vi "Process.vi"(8 "error in":errorcluster, 11 "Inst.Xeryon-Rotator":refnum<class "Inst.Xeryon-Rotator.lvclass">) -> (0 "error out":errorcluster, 3 "Inst.Xeryon-Rotator out":refnum<class "Inst.Xeryon-Rotator.lvclass">)   [LabVIEW 2019, in "Inst.Xeryon-Rotator.lvclass"]
doc: "---------------------------------------------------------------\nJKI State Machine Objects™\nhttp://jki.net/state-machine-objects/\nCopyright (C) 2005-2015, JKI <info@jki.net>\nALL RIGHTS RESERVED"
uses:
  Inst.Xeryon-Rotator.lvclass
  C:/Program Files/National Instruments/LabVIEW 2019/user.lib/LevyLab/Instrument Framework/Instrument Types/Cryostat/Instrument.Cryostat.lvclass
  C:/Program Files/National Instruments/LabVIEW 2019/user.lib/LevyLab/Instrument Framework/Instrument/Instrument.lvclass
  C:/Program Files/National Instruments/LabVIEW 2019/vi.lib/JKI/JKI SMO/SMO/SMO.lvclass
  <userlib>/LevyLab/Instrument Framework/Instrument/Instrument.lvclass
  <userlib>/LevyLab/RemoteControl/RemoteControl/Typedefs/Message--Cluster.ctl
  <userlib>/LevyLab/RemoteControl/RemoteControl/RemoteControl.lvclass
  Typedefs/PrivateEvents--Inst.Xeryon-Rotator.MessageToProcess.ctl
  f3e0a8c3-f545-4415-8120-73ea4d9772d3.vi
  cbce47eb-2e04-4774-9aae-1c3eb2914706.vi
  <vilib>/JDP Science/JSONtext/JSONtext.lvlib
  828899be-930a-4dca-b584-bfe75166f4b0.vi
  Typedefs/Inst.Xeryon-Rotator.ScanState--Enum.ctl
  <userlib>/LevyLab/Debug/Debug.lvlib
  <userlib>/LevyLab/Instrument Framework/Instrument Types/Cryostat/Typedefs/setAngle--cluster.ctl
  <userlib>/LevyLab/Instrument Framework/Instrument Types/Cryostat/Instrument.Cryostat.lvclass
  <userlib>/LevyLab/Instrument Framework/Instrument/API/Instrument.sendMessageToProcess (variant).vi
  <vilib>/JKI/JKI SMO/SMO/SMO.lvclass
  bd7500a4-fca6-4b1e-8595-4df63a7e1bab.vi
panel:
  out "Data":string
  out "Status":string
  out "State History":string
  # "Instrument.Xeryon-Rotator"
  # "Xeryon-Rotator"
  # "For instructions on how to use the JKI State Machine Objects, examples and video tutorials, visit:\nhttp://jki.net/state-machine-objects/\n\nJKI State Machine Objects™\nhttp://jki.net/state-machine-objects/\nCopyright (C) 2005-2015, JKI <info@jki.net>\nALL RIGHTS RESERVED"
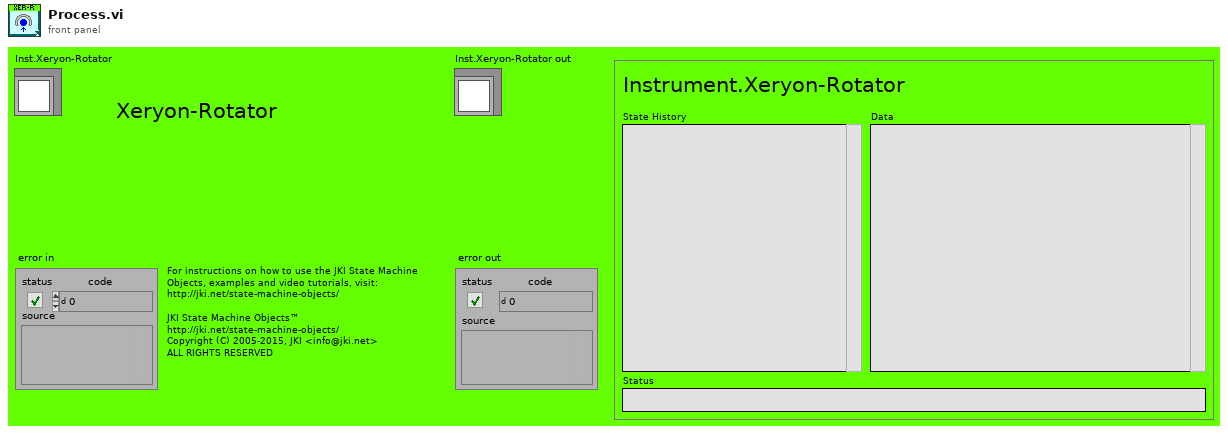
[diagram p1: front panel]
types:
  T1 = enum32{"invalid app kind", "Development System", "Run Time System", "Student Edition", "Embedded LabVIEW", "Evaluation", "Custom"}
  T2 = enum32{"Invalid", "Standard", "Closed", "Hidden", "Minimized", "Maximized"}
  T3 = typedef "Instrument.Cryostat.lvclass/setAngle--cluster.ctl" = cluster{"angle":dbl, "rate":dbl, "channel":i32}
  T4 = typedef "Inst.Xeryon-Rotator.lvclass/Inst.Xeryon-Rotator.ScanState--Enum.ctl" = enum16{"Scan Left", "Stop", "Scan Right", "Reset"}
  T5 = typedef "RemoteControl.lvlib/RemoteControl.lvclass/Message--Cluster.ctl" = cluster{"Command":string, "Data":variant, "ID":string, "error":errorcluster}
  T6 = typedef "Inst.Xeryon-Rotator.lvclass/PrivateEvents--Inst.Xeryon-Rotator.MessageToProcess.ctl" = cluster{"Message":T5}
  T7 = cluster{"Core":cluster{"Current VI Reference":refnum<vi>, "Close Panel on Exit?":bool, "Last Error":cluster{"error":errorcluster, "previous state":string, "remaining states":string}, "Shutdown?":bool}, "SMO":refnum<class "Inst.Xeryon-Rotator.lvclass">, "Running Step":i32, "sequence":string[], "MessageToProcess":T6}
  T8 = cluster{"Current VI Reference":refnum<vi>, "Close Panel on Exit?":bool, "Last Error":cluster{"error":errorcluster, "previous state":string, "remaining states":string}, "Shutdown?":bool}
  T9 = typedef "Debug.lvlib/Attribute.Debug.lvclass/DebugBehavior.ctl" = enum16{"Normal", "Debug"}
  T10 = typedef "SMO.lvclass/Protected Events.ctl" = cluster{"StopProcesses":refnum<user-event>, "AbortProcesses":refnum<user-event>, "Config Changed":refnum<user-event>, "Dependency":refnum<user-event>}
  T11 = cluster{"Encoder position [selected units]":dbl, "Desired Position [selected units]":dbl, "Status":string}
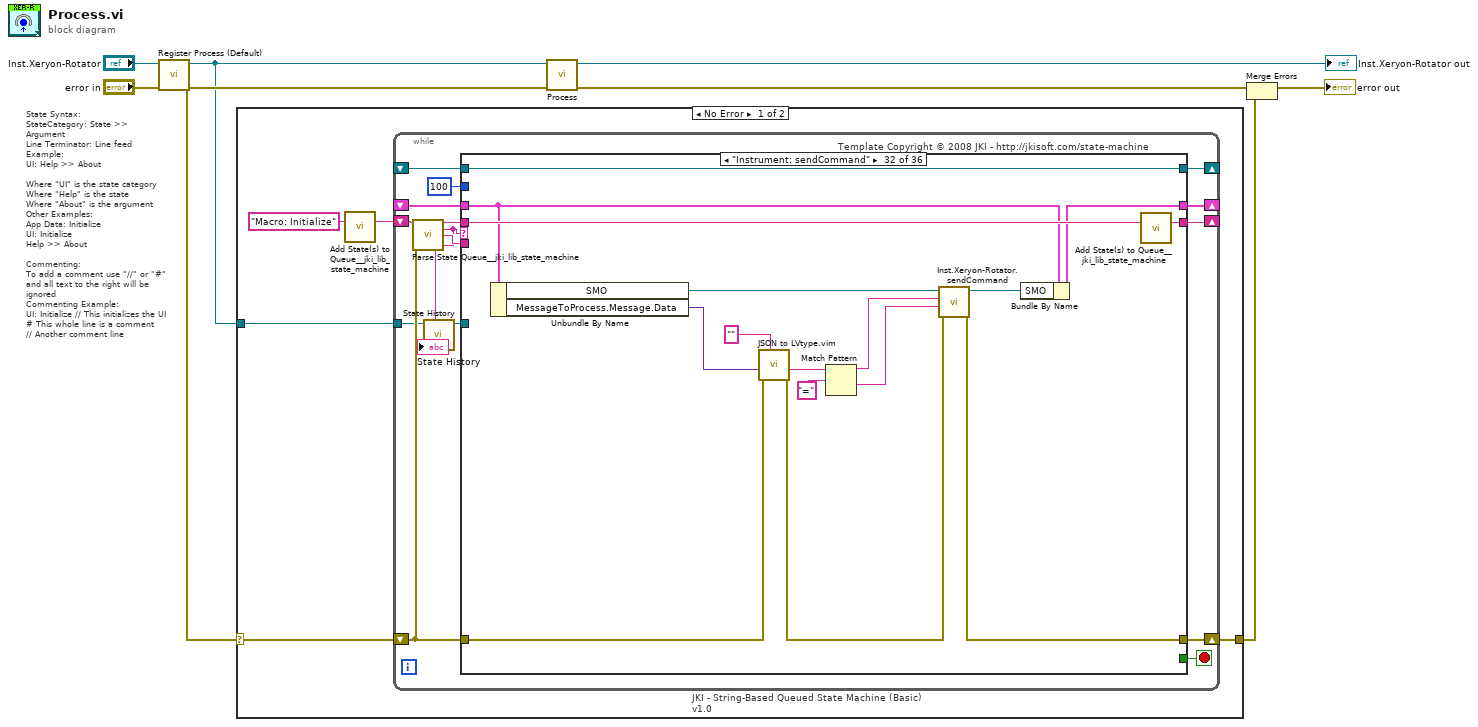
[diagram p0: block diagram]
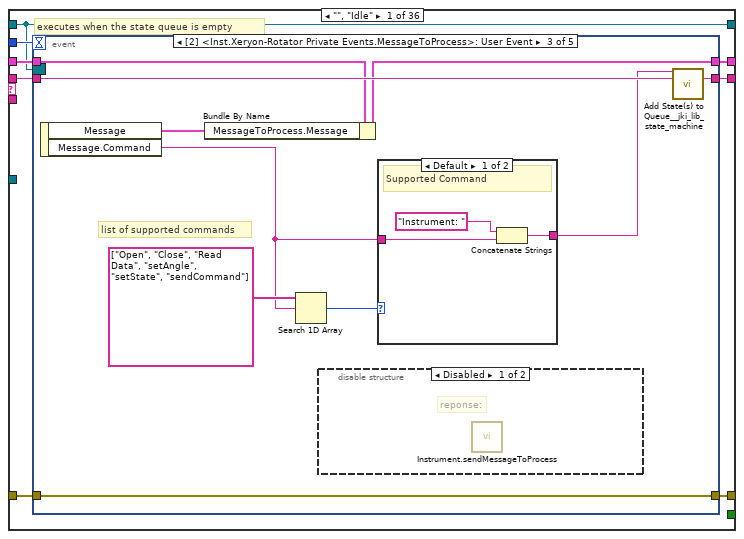
[diagram p2: hidden frame]
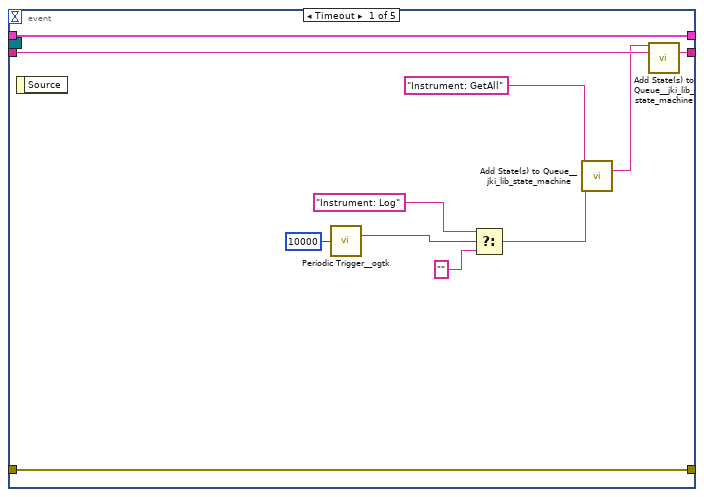
[diagram p3: hidden frame]
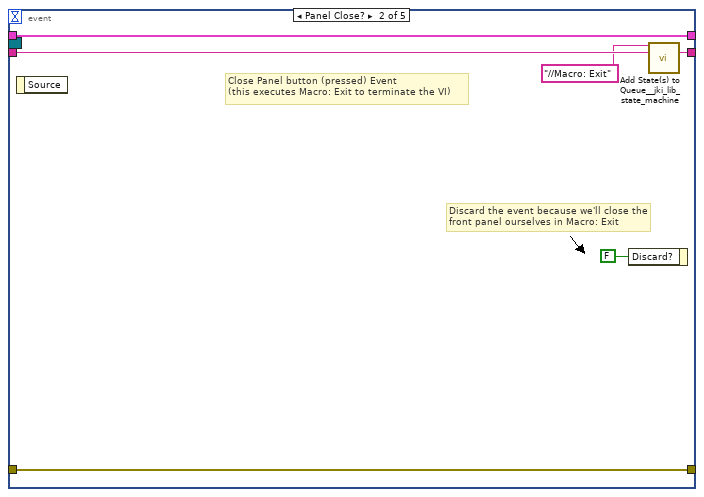
[diagram p4: hidden frame]
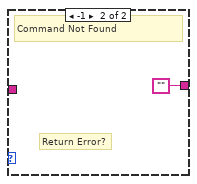
[diagram p6: hidden frame]
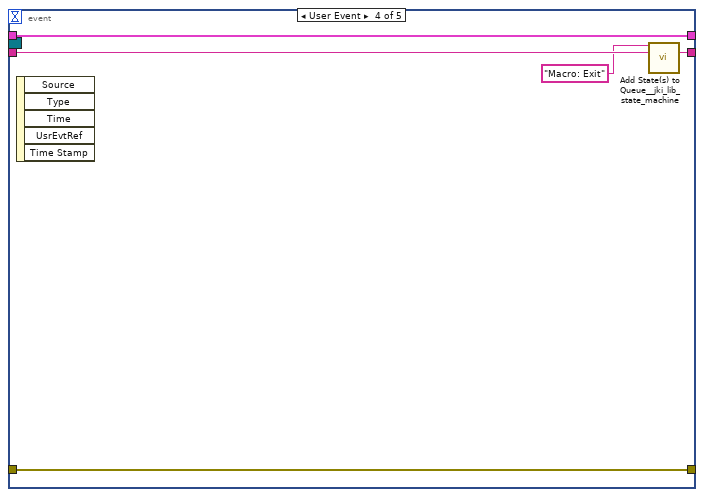
[diagram p7: hidden frame]
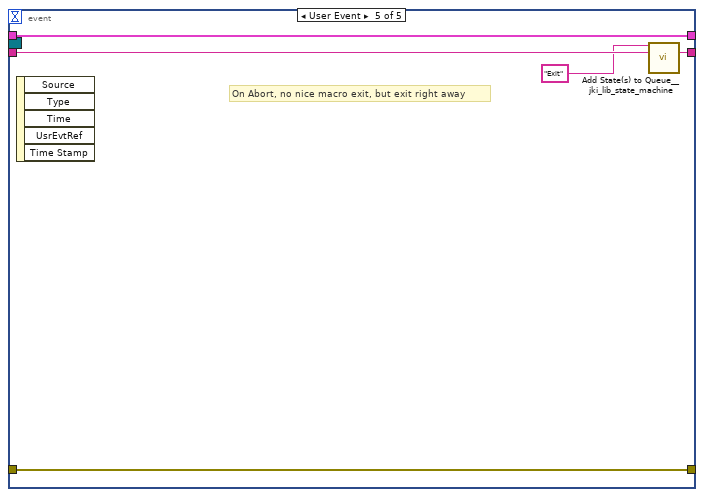
[diagram p8: hidden frame]
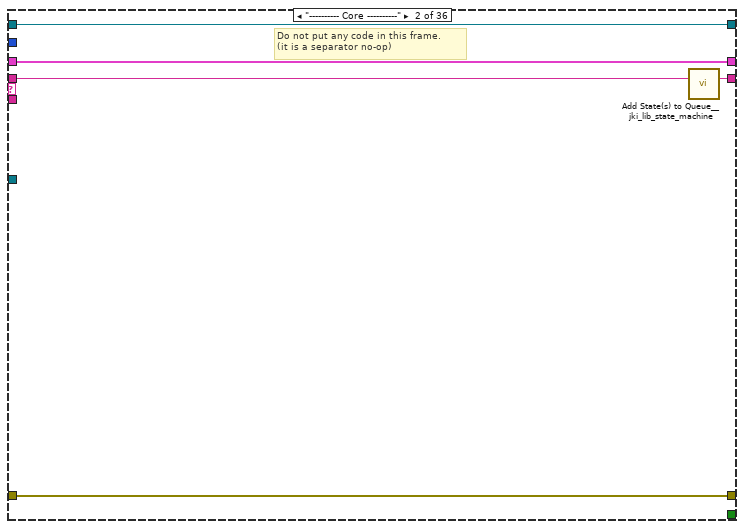
[diagram p9: hidden frame]
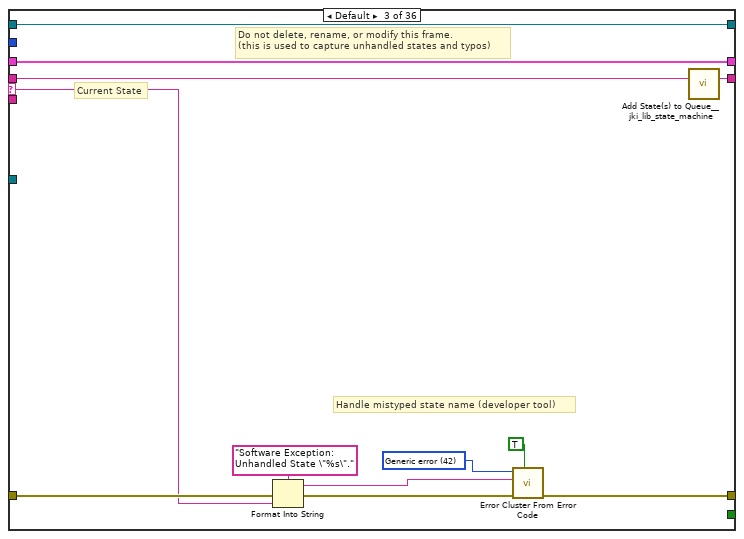
[diagram p10: hidden frame]
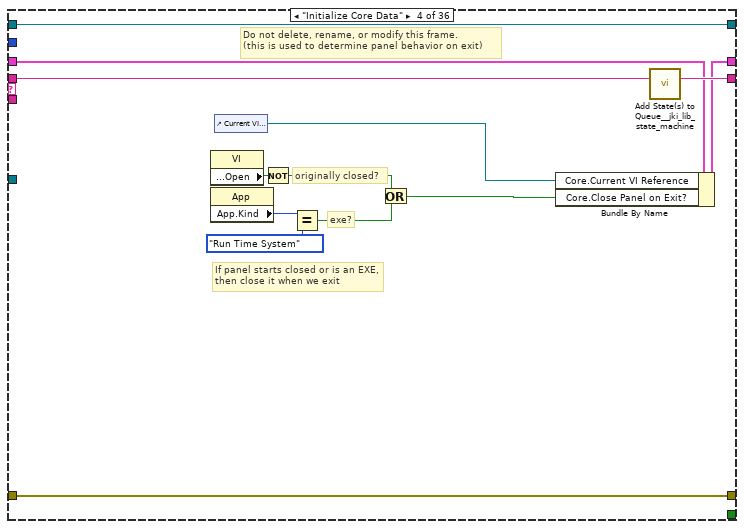
[diagram p11: hidden frame]
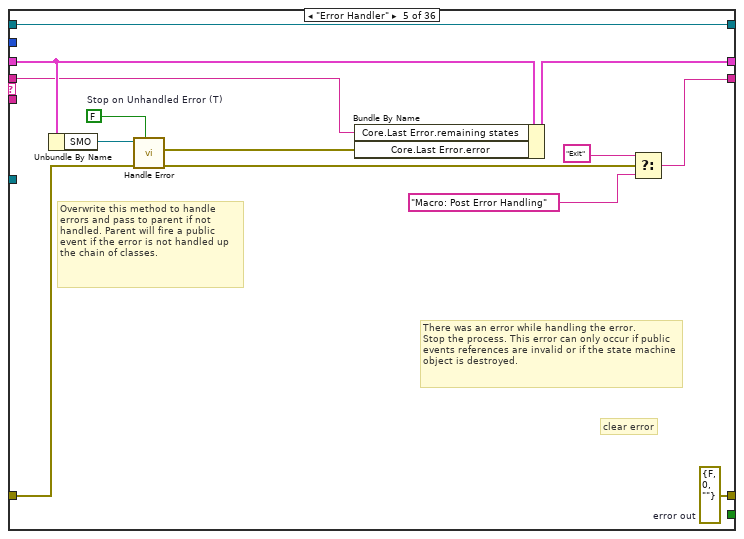
[diagram p12: hidden frame]
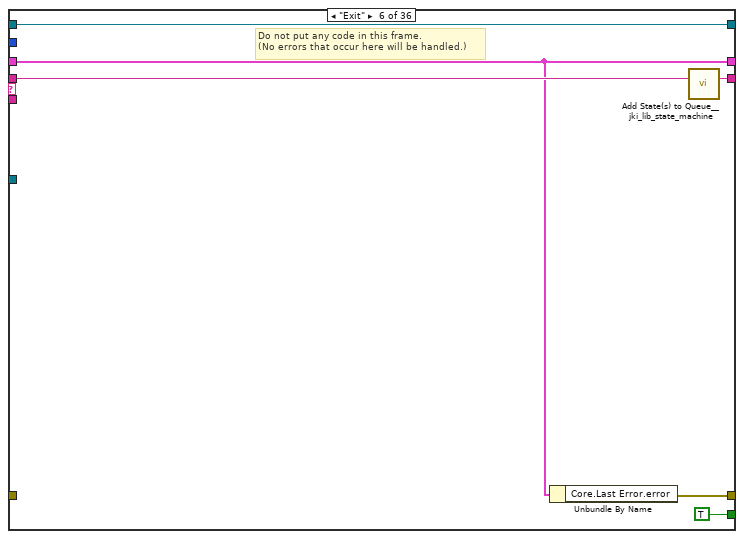
[diagram p13: hidden frame]
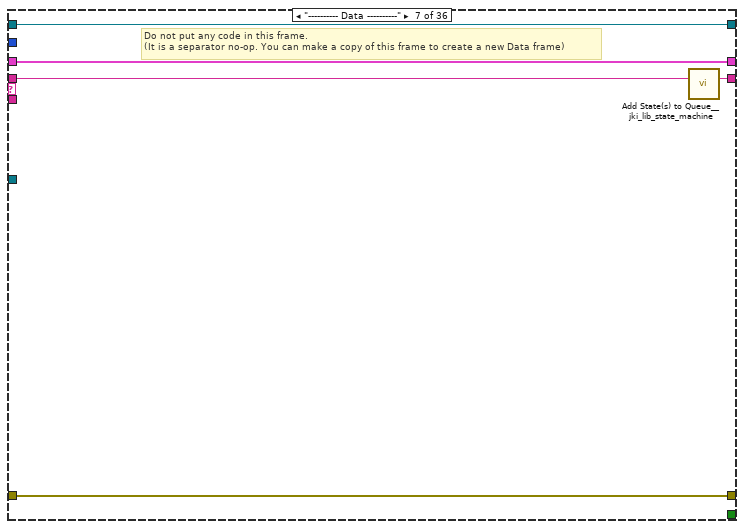
[diagram p14: hidden frame]
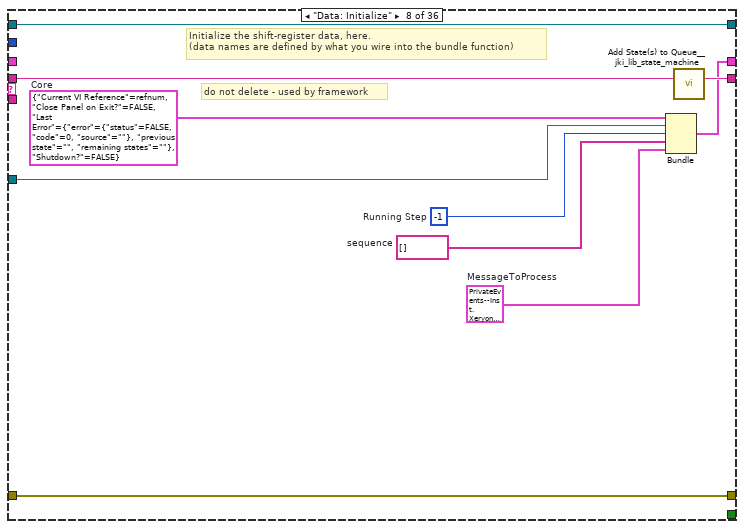
[diagram p15: hidden frame]
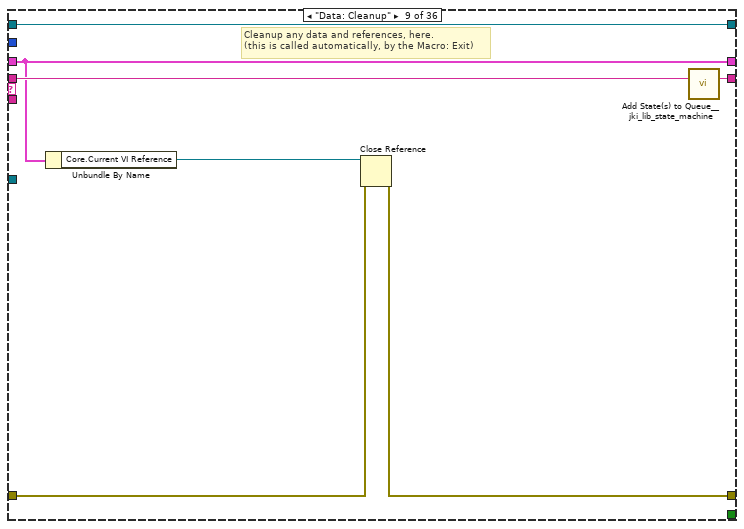
[diagram p16: hidden frame]
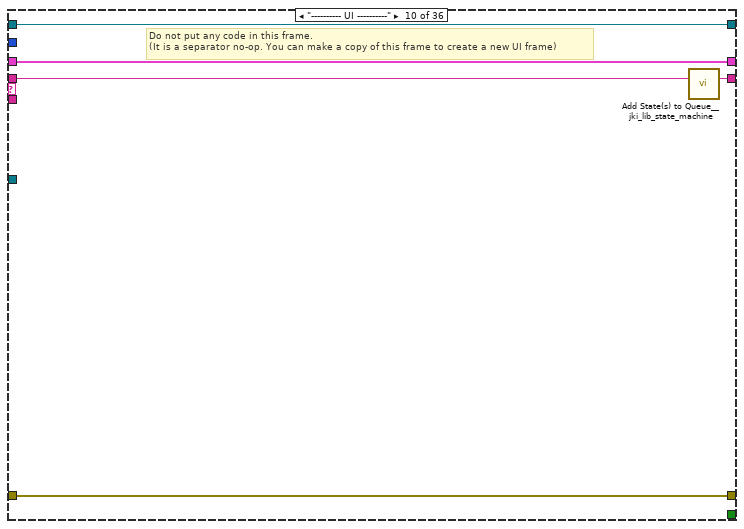
[diagram p17: hidden frame]
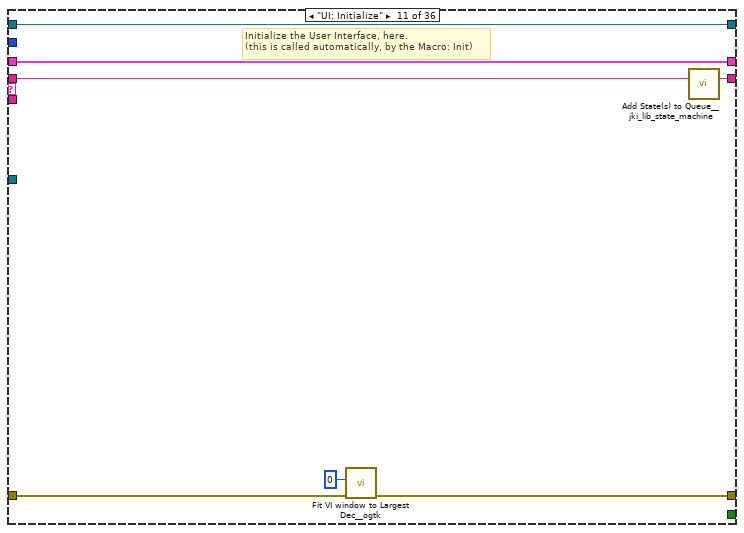
[diagram p18: hidden frame]
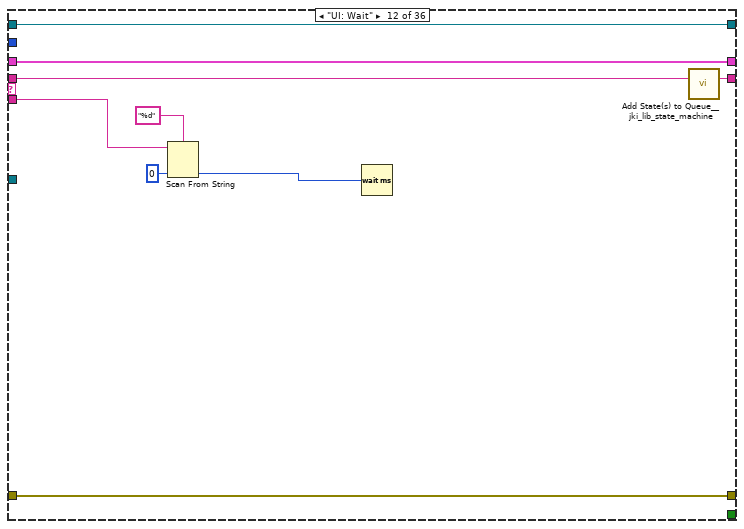
[diagram p19: hidden frame]
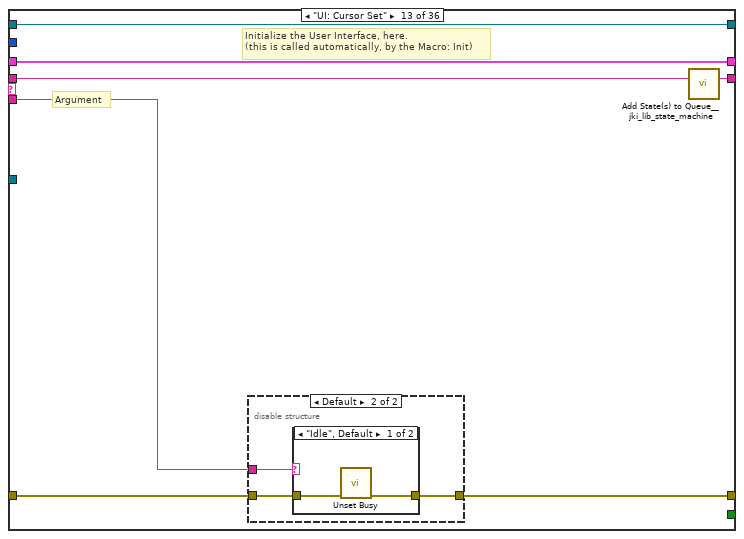
[diagram p20: hidden frame]
diagram:
  # "State Syntax:\nStateCategory: State >> Argument\nLine Terminator: Line feed\nExample:\nUI: Help >> About\n\nWhere \"UI\" is the state category\nWhere \"Help\" is the state\nWhere \"About\" is the argument\nOther Examples:\nApp Data: Initialize\nUI: Initialize\nHelp >> About\n\nCommenting:\nTo add a comment use \"//\" or \"#\" and all text to the right will be ignored\nCommenting Example:\nUI: Initialize // This initializes the UI\n# This whole line is a comment\n// Another comment line"
  n1 = call <vilib>:"Register Process (Default).vi"("error in (no error)"="error in", "SMO"="Inst.Xeryon-Rotator") -> ("error out"=w5:errorcluster, "SelfRef"=w4:refnum<class "Inst.Xeryon-Rotator.lvclass">)  [unwired: 8 in]
  n2 = case shown="No Error" w5 {
    selector: w5 -> [w10 w485]
    tunnel: w4 -> [w11 _]
    tunnel: [w9 w485] -> w1
    frame No Error {
      n3 = call <vilib>:"Add State(s) to Queue__jki_lib_state_machine.vi"("State(s) in (\"\")"="Macro: Initialize") -> ("States Out"=w13:string)  [unwired: 14 in]
      n4 = while "JKI - String-Based Queued State Machine (Basic) v1.0" {
        shift-right: [w23] -> _
        shift-left: _ -> [w22]
        shift-right: [w26] -> w9
        shift-left: w10 -> [w20]
        shift-right: [w25] -> _
        shift-left: w13 -> [w27]
        tunnel: w11 -> [w14]
        shift-right: [w19] -> _
        shift-left: _ -> [w18]
        stop <- w24 stop-if-true
        # "Template Copyright © 2008 JKI - http://jkisoft.com/state-machine"
        n5 = call <vilib>:"Parse State Queue__jki_lib_state_machine.vi"("State Queue"=w27, "Error In (no error)"=w20) -> ("Remaining States"=w29:string, "Current State"=w17:string, "Arguments"=w28:string)  [unwired: 11 in]
        n6 = call <userlib>:"State History.vi"("Current State"=w17, "SMO"=w14) -> ("SMO"=w15:refnum<class "Inst.Xeryon-Rotator.lvclass">, "History"=→"State History":string)  [unwired: 8 in]
        n7 = case shown="\"Instrument: sendCommand\"" w17 {
          selector: w17 -> [_ _ w85 _ _ _ _ _ _ _ _ _ _ _ _ _ _ _ _ _ _ _ _ _ _ _ _ _ _ _ _ _ _ _ _ _]
          tunnel: w29 -> [w37 w83 w89 w108 w113 w127 w132 w142 w149 w154 w161 w170 w177 w193 w225 w234 w249 w266 w287 w304 w309 w320 w325 w338 w344 w351 w360 w369 w383 w409 w422 w438 w454 w459 w465 w484]
          tunnel: w28 -> [_ _ _ _ _ _ _ _ _ _ _ w162 w171 w187 _ _ _ _ _ _ _ _ _ _ _ _ _ _ _ _ _ _ _ _ w460 w468]
          tunnel: w22 -> [w35 w80 w87 w99 w117 w123 w129 _ w144 w151 w159 w167 w175 w189 w222 w231 w236 w256 w277 w291 w306 w317 w322 w331 w342 w346 w356 w365 w379 w405 w418 w434 w450 w455 w461 w474]
          tunnel: [w34 w81 w91 w105 w118 w122 w130 w134 w145 w152 w156 w168 w172 w190 w223 w226 w239 w264 w285 w293 w307 w311 w323 w334 w340 w348 w353 w362 w374 w404 w415 w427 w446 w456 w462 w476] -> w26
          tunnel: w20 -> [w33 w81 w90 w105 w119 _ w130 w134 w146 w152 w155 w168 w173 w191 w223 w226 w238 w264 w285 w293 w307 w312 w323 w328 w340 w348 w352 w361 w377 w393 w412 w432 w449 w456 w462 w470]
          tunnel: [w36 w82 w88 w107 w109 w126 w131 w141 w148 w153 w160 w169 w176 w192 w224 w233 w248 w265 w286 w303 w308 w319 w324 w337 w343 w350 w359 w368 w382 w408 w421 w437 w453 w458 w464 w483] -> w25
          tunnel: [_ _ _ _ _ TRUE _ _ _ _ _ _ _ _ _ _ _ _ _ _ _ _ _ _ _ _ _ _ _ _ _ _ _ _ _ _] -> w24
          tunnel: [w32 w80 w87 w106 w116 w123 w129 w140 w144 w151 w159 w167 w175 w189 w222 w231 w237 w257 w278 w288 w306 w317 w322 w331 w342 w347 w357 w366 w380 w406 w419 w435 w451 w455 w461 w473] -> w23
          tunnel: 100 ("Timeout") -> [w31 _ _ _ _ _ _ _ _ _ _ _ _ _ _ _ _ _ _ _ _ _ _ _ _ _ _ _ _ _ _ _ _ _ _ _]
          tunnel: w15 -> [_ _ _ _ _ _ _ w135 _ _ _ _ _ _ _ _ _ _ _ _ _ _ _ _ _ _ _ _ _ _ _ _ _ _ _ _]
          tunnel: [w30 w79 w84 w96 w121 w124 w128 w139 w143 w150 w158 w166 w174 w186 w221 w232 w247 w263 w284 w299 w305 w318 w321 w336 w341 w349 w358 w367 w381 w407 w420 w436 w452 w457 w463 w482] -> w19
          tunnel: w18 -> [w30 w79 w84 w96 w121 w124 w128 w139 w143 w150 w158 w166 w174 w186 w221 w232 w247 w263 w284 w299 w305 w318 w321 _ w341 w349 w358 w367 w381 w407 w420 w436 w452 w457 w463 w482]
          frame "", "Idle" {
            # "executes when the state queue is empty"
            n8 = event shown="[2] <Inst.Xeryon-Rotator Private Events.MessageToProcess>: User Event" {
              selector: w30 -> [_ _ _ _ _]
              dyn-events: _ -> [_ _ _ _ _]
              timeout: w31 -> [_ _ _ _ _]
              tunnel: w37 -> [w48 w54 w64 w73 w78]
              tunnel: [w47 w53 w63 w72 w77] -> w36
              tunnel: w35 -> [w45 w51 w56 w70 w75]
              tunnel: [w46 w52 w62 w71 w76] -> w34
              tunnel: w33 -> [w46 w52 w62 w71 w76]
              tunnel: [w45 w51 w57 w70 w75] -> w32
              event Timeout {
                n9 = event-data() -> ()  [unwired: 1 in, 1 out]
                n10 = call <userlib>:"Periodic Trigger__ogtk.vi"("time (ms)"=u32 10000) -> ("Triggered"=w42:bool)  [unwired: 12 in, 2 out]
                n11 = Select(t="Instrument: Log" ("State(s) in Front (\"\")"), s=w42, f="") -> (s? t:f=w41:string)
                n12 = call <vilib>:"Add State(s) to Queue__jki_lib_state_machine.vi"("State(s) in Front (\"\")"="Instrument: GetAll" ("State(s) in Front (\"\")"), "State(s) at Back (\"\")"=w41) -> ("States Out"=w39:string)  [unwired: 13 in]
                n13 = call <vilib>:"Add State(s) to Queue__jki_lib_state_machine.vi"("State(s) in Front (\"\")"=w39, "State(s) in (\"\")"=w48) -> ("States Out"=w47:string)  [unwired: 13 in]
              }
              event Panel Close? {
                # "Discard the event because we'll close the front panel ourselves in Macro: Exit"
                # "Close Panel button (pressed) Event\n(this executes Macro: Exit to terminate the VI)"
                n14 = event-data() -> ()  [unwired: 1 in, 1 out]
                n15 = event-data("Discard?"=FALSE) -> ()  [unwired: 1 in, 1 out]
                n16 = call <vilib>:"Add State(s) to Queue__jki_lib_state_machine.vi"("State(s) in Front (\"\")"="//Macro: Exit", "State(s) in (\"\")"=w54) -> ("States Out"=w53:string)  [unwired: 13 in]
              }
              event User Event {
                # "list of supported commands"
                n17 = event-data() -> ("Message"=w55:T5, "Message.Command"=w58:string)  [unwired: 1 in]
                n18 = Bundle By Name(cluster=w56, "MessageToProcess.Message"=w55) -> (w57:T7)
                n19 = Search 1D Array(1D array=string[] ["Open", "Close", "Read Data", "setAngle", "setState", "sendCommand"], element=w58) -> (index of element=w61:i32)  [unwired: 1 in]
                n20 = disable-structure shown="Disabled" {
                  frame Disabled {
                    # "reponse:"
                    n21 = call-poly <userlib>:"Instrument.sendMessageToProcess.vi"() -> ()  [unwired: 10 in, 2 out]
                  }
                  frame Enabled {
                  }
                }
                n22 = case shown="Default" w61 {
                  tunnel: [w67 "" ("Empty String Constant")] -> w59
                  tunnel: w58 -> [w66 _]
                  frame Default {
                    # "Supported Command"
                    n23 = Concatenate Strings("Instrument: ", w66) -> (w67:string)
                  }
                  frame -1 {
                    # "Return Error?"
                    # "Command Not Found"
                  }
                }
                n24 = call <vilib>:"Add State(s) to Queue__jki_lib_state_machine.vi"("State(s) in Front (\"\")"=w59, "State(s) in (\"\")"=w64) -> ("States Out"=w63:string)  [unwired: 13 in]
              }
              event User Event {
                n25 = event-data() -> ()  [unwired: 1 in, 5 out]
                n26 = call <vilib>:"Add State(s) to Queue__jki_lib_state_machine.vi"("State(s) in Front (\"\")"="Macro: Exit", "State(s) in (\"\")"=w73) -> ("States Out"=w72:string)  [unwired: 13 in]
              }
              event User Event {
                # "On Abort, no nice macro exit, but exit right away"
                n27 = event-data() -> ()  [unwired: 1 in, 5 out]
                n28 = call <vilib>:"Add State(s) to Queue__jki_lib_state_machine.vi"("State(s) in Front (\"\")"="Exit", "State(s) in (\"\")"=w78) -> ("States Out"=w77:string)  [unwired: 13 in]
              }
            }
          }
          frame "---------- Core ----------" {
            # "Do not put any code in this frame.\n(it is a separator no-op)"
            n29 = call <vilib>:"Add State(s) to Queue__jki_lib_state_machine.vi"("State(s) in (\"\")"=w83) -> ("States Out"=w82:string)  [unwired: 14 in]
          }
          frame Default {
            w94 = 42 items=["No error", "Argument error", "Memory is full", "Out of zone", "End of file", "File already open", "Generic file I/O error", "File not found", "File permission error", "Disk is full", "Duplicate path", "Too many files open", "System feature not enabled", "Resource file not found", "Cannot add resource", "Resource not found", "Image not found", "Image memory error", "Pen does not exist", "Config type invalid", "Config token not found", "Config parse error", "Config memory error", "Bad external code format", "Bad external code offset", "External code not present", "Null window", "Destroy window error", "Null menu", "Print aborted", "Bad print record", "Print driver error", "Windows error during printing", "Memory error during printing", "Print dialog error", "Generic print error", "Invalid device refnum", "Device not found", "Device parameter error", "Device unit error", "Cannot open device", "Device call aborted", "Generic error", "Cancelled by user", "Object ID too low", "Object ID too high", "Object not in heap", "Unknown heap", "Unknown object (invalid DefProc)", "Unknown object (DefProc not in table)", "Message out of range", "Invalid (null) method", "Unknown message", "Manager call not supported", "Bad address", "Network operation in progress", "Network operation timed out", "Connection is busy", "Network attribute not supported", "Network error", "Address in use", "System out of memory", "Connection aborted", "Connection refused", "Not connected", "Already connected", "Connection closed", "Initialization error (interapplication manager)", "Bad occurrence", "Wait on unbound occurrence handler", "Occurrence queue overflow", "Datalog type conflict", "Unused", "Unrecognized type (interapplication manager)", "Memory corrupt", "Failed to make temporary DLL", "Old CIN version", "Drag socket not found", "Failed to load drop-object", "Failed to register OLE object", "Failed to release OLE object", "Format specifier type mismatch", "Unknown format specifier", "Too few format specifiers", "Too many format specifiers", "Scan failed", "Newer CIN version", "Error converting to variant", "Runtime menu error", "Password tampered", "Variant attribute not found", "Incompatible variant data type", "Event data is not available", "Event Store is not present", "Occurrence is not found", "Event Queue is not created", "Event info is not available", "Refnum passed is NULL", "Error retrieving Class GUID", "Error retrieving CoClass GUID", "Error retrieving TypeLib GUID.", "Bad built application magic bytes.", "Specific driver is different from the specific driver associated with the Logical Name.", "There is no session opened to the class driver.", "Max Error", "MAX - Error with config objects", "MAX - Error loading configuration", "MAX - Group not supported"]
            # "Current State"
            # "Do not delete, rename, or modify this frame.\n(this is used to capture unhandled states and typos)"
            # "Handle mistyped state name (developer tool)"
            n30 = Format Into String(format string="Software Exception: Unhandled State \"%s\"." ("message"), error in=w90, w85) -> (resulting string=w93:string, error out=w92:errorcluster)  [unwired: 1 in]
            n31 = call <vilib>:"Error Cluster From Error Code.vi"("show call chain? (False)"=TRUE, "error in (no error)"=w92, "error message (\"\")"=w93, "error code (0)"=w94) -> ("error out"=w91:errorcluster)  [unwired: 5 in]
            n32 = call <vilib>:"Add State(s) to Queue__jki_lib_state_machine.vi"("State(s) in (\"\")"=w89) -> ("States Out"=w88:string)  [unwired: 14 in]
          }
          frame "Initialize Core Data" {
            # "Do not delete, rename, or modify this frame.\n(this is used to determine panel behavior on exit)"
            # "originally closed?"
            # "exe?"
            # "If panel starts closed or is an EXE, then close it when we exit"
            n33 = property class="VI"() -> ("Front Panel.Open"=w104:bool)  [unwired: 2 in, 2 out]
            n34 = property class="App"() -> ("App.Kind"=w103:T1)  [unwired: 2 in, 2 out]
            n35 = control-ref of="Current VI Reference"() -> (w97:refnum<vi>)
            n36 = Not(x=w104) -> (.not. x?=w101:bool)
            n37 = Equal?(x=w103, y=T1."Run Time System" ("Application:Kind")) -> (x = y?=w100:bool)
            n38 = Or(x=w101, y=w100) -> (x .or. y?=w98:bool)
            n39 = Bundle By Name(cluster=w99, "Core.Current VI Reference"=w97, "Core.Close Panel on Exit?"=w98) -> (w106:T7)
            n40 = call <vilib>:"Add State(s) to Queue__jki_lib_state_machine.vi"("State(s) in (\"\")"=w108) -> ("States Out"=w107:string)  [unwired: 14 in]
          }
          frame "Error Handler" {
            w114 = FALSE  # Stop on Unhandled Error (T)
            w118 = errorcluster {"status"=FALSE, "code"=0, "source"=""}  # error out
            # "clear error"
            # "There was an error while handling the error.\nStop the process. This error can only occur if public events references are invalid or if the state machine object is destroyed."
            # "Overwrite this method to handle errors and pass to parent if not handled. Parent will fire a public event if the error is not handled up the chain of classes."
            n41 = Unbundle By Name(w117) -> ("SMO"=w120:refnum<class "Inst.Xeryon-Rotator.lvclass">)
            n42 = call-dynamic "Handle Error.vi"("Stop on Unhandled Error (T)"=w114, "error in"=w119, "SMO"=w120) -> ("handling error"=w110:errorcluster, "Unhandled error"=w115:errorcluster)  [unwired: 6 in, 1 out]
            n43 = Bundle By Name(cluster=w117, "Core.Last Error.remaining states"=w113, "Core.Last Error.error"=w115) -> (w116:T7)
            n44 = Select(t="Exit", s=w110, f="Macro: Post Error Handling") -> (s? t:f=w109:string)
          }
          frame "Exit" {
            # "Do not put any code in this frame.\n(No errors that occur here will be handled.)"
            n45 = Unbundle By Name(w123) -> ("Core.Last Error.error"=w122:errorcluster)
            n46 = call <vilib>:"Add State(s) to Queue__jki_lib_state_machine.vi"("State(s) in (\"\")"=w127) -> ("States Out"=w126:string)  [unwired: 14 in]
          }
          frame "---------- Data ----------" {
            # "Do not put any code in this frame.\n(It is a separator no-op. You can make a copy of this frame to create a new Data frame)"
            n47 = call <vilib>:"Add State(s) to Queue__jki_lib_state_machine.vi"("State(s) in (\"\")"=w132) -> ("States Out"=w131:string)  [unwired: 14 in]
          }
          frame "Data: Initialize" {
            w133 = T6 {"Message"={"Command"="", "Data"=variant(string ""), "ID"="", "error"={"status"=FALSE, "code"=0, "source"=""}}}  # MessageToProcess
            w136 = string[] []  # sequence
            w137 = -1  # Running Step
            w138 = T8 {"Current VI Reference"=refnum, "Close Panel on Exit?"=FALSE, "Last Error"={"error"={"status"=FALSE, "code"=0, "source"=""}, "previous state"="", "remaining states"=""}, "Shutdown?"=FALSE}  # Core
            # "do not delete - used by framework"
            # "Initialize the shift-register data, here.\n(data names are defined by what you wire into the bundle function)"
            n48 = Bundle("Core"=w138, "SMO"=w135, "Running Step"=w137, "sequence"=w136, "MessageToProcess"=w133) -> (w140:T7)  [unwired: 1 in]
            n49 = call <vilib>:"Add State(s) to Queue__jki_lib_state_machine.vi"("State(s) in (\"\")"=w142) -> ("States Out"=w141:string)  [unwired: 14 in]
          }
          frame "Data: Cleanup" {
            # "Cleanup any data and references, here.\n(this is called automatically, by the Macro: Exit)"
            n50 = Unbundle By Name(w144) -> ("Core.Current VI Reference"=w147:refnum<vi>)
            n51 = Close Reference(reference=w147, error in (no error)=w146) -> (error out=w145:errorcluster)
            n52 = call <vilib>:"Add State(s) to Queue__jki_lib_state_machine.vi"("State(s) in (\"\")"=w149) -> ("States Out"=w148:string)  [unwired: 14 in]
          }
          frame "---------- UI ----------" {
            # "Do not put any code in this frame.\n(It is a separator no-op. You can make a copy of this frame to create a new UI frame)"
            n53 = call <vilib>:"Add State(s) to Queue__jki_lib_state_machine.vi"("State(s) in (\"\")"=w154) -> ("States Out"=w153:string)  [unwired: 14 in]
          }
          frame "UI: Initialize" {
            # "Initialize the User Interface, here.\n(this is called automatically, by the Macro: Init)"
            n54 = call <userlib>:"Fit VI window to Largest Dec__ogtk.vi"("error in (no error)"=w155, "border spacing (2 px)"=0) -> ("error out"=w156:errorcluster)  [unwired: 4 in, 1 out]
            n55 = call <vilib>:"Add State(s) to Queue__jki_lib_state_machine.vi"("State(s) in (\"\")"=w161) -> ("States Out"=w160:string)  [unwired: 14 in]
          }
          frame "UI: Wait" {
            n56 = Scan From String(format string="%d", input string=w162, default 1=u32 0 ("default value 1")) -> (output 1=w163:u32)  [unwired: 2 in, 3 out]
            n57 = Wait (ms)(milliseconds to wait=w163) -> ()  [unwired: 1 out]
            n58 = call <vilib>:"Add State(s) to Queue__jki_lib_state_machine.vi"("State(s) in (\"\")"=w170) -> ("States Out"=w169:string)  [unwired: 14 in]
          }
          frame "UI: Cursor Set" {
            # "Argument"
            # "Initialize the User Interface, here.\n(this is called automatically, by the Macro: Init)"
            n59 = disable-structure shown="Default" {
              disable-tunnel: w173 -> [w178 w181]
              disable-tunnel: [w178 w180] -> w172
              disable-tunnel: w171 -> [_ w179]
              frame condition #0 {
              }
              frame condition #1 (active) {
                n60 = case shown="\"Idle\", Default" w179 {
                  tunnel: w181 -> [w183 w185]
                  tunnel: [w182 w184] -> w180
                  frame "Idle", Default {
                    n61 = call <vilib>:"Unset Busy.vi"("error in (no error)"=w183) -> ("error out"=w182:errorcluster)  [unwired: 10 in]
                  }
                  frame "Busy" {
                    n62 = call <vilib>:"Set Busy.vi"("error in (no error)"=w185) -> ("error out"=w184:errorcluster)  [unwired: 9 in, 1 out]
                  }
                }
              }
            }
            n63 = call <vilib>:"Add State(s) to Queue__jki_lib_state_machine.vi"("State(s) in (\"\")"=w177) -> ("States Out"=w176:string)  [unwired: 14 in]
          }
          frame "UI: Front Panel State" {
            # "Argument"
            # "Set Front Panel Open or Closed\n(Usage: \"UI: Front Panel State >> Open|Close\")"
            n64 = Unbundle By Name(w189) -> ("Core.Current VI Reference"=w188:refnum<vi>)
            n65 = disable-structure shown="TARGET_TYPE==RT" {
              disable-tunnel: w191 -> [w197 w220]
              disable-tunnel: [w196 w220] -> w190
              disable-tunnel: w188 -> [w195 _]
              disable-tunnel: w187 -> [w194 _]
              frame condition #0 (active) {
                n66 = case shown="\"Close\"" w194 {
                  tunnel: w197 -> [w201 w214]
                  tunnel: [w203 w215] -> w196
                  tunnel: w195 -> [w202 w212]
                  frame "Open", Default {
                    n67 = property class="VI"(reference=w202, error in=w201) -> (reference out=w199:refnum<vi>, error out=w200:errorcluster, "FP.State"=w198:T2)
                    n68 = case shown="\"Closed\"" w198 {
                      tunnel: [w206 w209] -> w203
                      tunnel: w200 -> [w205 w209]
                      tunnel: w199 -> [w204 _]
                      frame "Closed" {
                        n69 = invoke class="VI" method="FP.Open"(reference=w204, error in=w205, "Activate"=TRUE, "State"=T2."Standard") -> (error out=w206:errorcluster)  [unwired: 1 in, 4 out]
                      }
                      frame Default {
                      }
                    }
                  }
                  frame "Close" {
                    n70 = property class="VI"(reference=w212, error in=w214) -> (reference out=w211:refnum<vi>, error out=w213:errorcluster, "FP.State"=w210:T2)
                    n71 = case shown="Default" w210 {
                      tunnel: [w216 w219] -> w215
                      tunnel: w213 -> [w216 w218]
                      tunnel: w211 -> [_ w217]
                      frame "Invalid", "Closed" {
                      }
                      frame Default {
                        n72 = invoke class="VI" method="FP.Close"(reference=w217, error in=w218) -> (error out=w219:errorcluster)  [unwired: 1 in, 2 out]
                      }
                    }
                  }
                }
              }
              frame condition #1 {
              }
            }
            n73 = call <vilib>:"Add State(s) to Queue__jki_lib_state_machine.vi"("State(s) in (\"\")"=w193) -> ("States Out"=w192:string)  [unwired: 14 in]
          }
          frame "---------- Macro ----------" {
            # "Do not put any code in this frame.\n(It is a separator no-op. You can make a copy of this frame to create a new Macro frame)"
            n74 = call <vilib>:"Add State(s) to Queue__jki_lib_state_machine.vi"("State(s) in (\"\")"=w225) -> ("States Out"=w224:string)  [unwired: 14 in]
          }
          frame "Macro: Initialize" {
            # "Initialization Macro\n(This is called once, when the VI starts)"
            n75 = call <vilib>:"Add State(s) to Queue__jki_lib_state_machine.vi"("State(s) in Front (\"\")"="Data: Initialize\nInitialize Core Data\nEvents: Register", "State(s) in (\"\")"="Process: Sync", "State(s) at Back (\"\")"="UI: Initialize\nUI: Front Panel State >> Close\nMacro: Debug\nInstrument: Open Hardware") -> ("States Out"=w229:string)  [unwired: 12 in]
            n76 = call <vilib>:"Add State(s) to Queue__jki_lib_state_machine.vi"("State(s) in Front (\"\")"=w229, "State(s) in (\"\")"=w234) -> ("States Out"=w233:string)  [unwired: 13 in]
          }
          frame "Macro: Debug" {
            # "exe?"
            # "If pane is an EXE, then close it when we exit"
            # "Macro: Debug\n(get debug behavior, determine UI and determine shutdown behavior)"
            n77 = Unbundle By Name(w236) -> ("Core.Close Panel on Exit?"=w241:bool, "SMO"=w246:refnum<class "Inst.Xeryon-Rotator.lvclass">)
            n78 = property class="App"() -> ("App.Kind"=w244:T1)  [unwired: 2 in, 2 out]
            n79 = Equal?(x=w244, y=T1."Run Time System" ("Application:Kind")) -> (x = y?=w240:bool)
            n80 = call <userlib>:"Get Debug Mode.vi"("error in (no error)"=w238, "SMO"=w246) -> ("error out"=w239:errorcluster, "Behavior"=w245:T9)  [unwired: 7 in, 1 out]
            n81 = case shown="\"Debug\"" w245 {
              tunnel: [w250 w252] -> w242
              tunnel: w241 -> [w250 _]
              tunnel: w240 -> [_ w254]
              tunnel: [_ "UI: Front Panel State >> Open\nUI: Wait >> 1000"] -> w235
              frame "Normal", Default {
                # "respect core.close"
              }
              frame "Debug" {
                # "keep panel open\nunless exe"
                n82 = Or(x=w254, y=FALSE) -> (x .or. y?=w252:bool)
              }
            }
            n83 = Bundle By Name(cluster=w236, "Core.Close Panel on Exit?"=w242) -> (w237:T7)
            n84 = call <vilib>:"Add State(s) to Queue__jki_lib_state_machine.vi"("State(s) in Front (\"\")"=w235, "State(s) in (\"\")"=w249) -> ("States Out"=w248:string)  [unwired: 13 in]
          }
          frame "Macro: Post Error Handling" {
            # "Clear Last Error?"
            n85 = Unbundle By Name(w256) -> ("Core.Last Error.remaining states"=w258:string, "Core.Shutdown?"=w259:bool)
            n86 = Unbundle By Name(w256) -> ("Core.Last Error.error"=w262:errorcluster)
            n87 = case shown="False" FALSE {
              tunnel: w262 -> [w270 _]
              tunnel: [w270 _] -> w261
              frame False {
              }
              frame True {
              }
            }
            n88 = case shown="True" w259 {
              tunnel: w258 -> [w267 w269]
              tunnel: [w267 w268] -> w255
              frame False {
                # "These are the remaining states (at the moment the error occured). States can be altered according to business logic."
                # "NOT SHUTTING DOWN"
              }
              frame True {
                # "Developer can decide to alter the states but should be aware that during the shutdown process, there are certain states that must be run for the SMO to properly shut itself (and this process) down. As such, one can add states to perform additional clean-ups, but should append the remaining state to be executed."
                # "SHUTTING DOWN"
                n89 = call <vilib>:"Add State(s) to Queue__jki_lib_state_machine.vi"("State(s) in (\"\")"=w269) -> ("States Out"=w268:string)  [unwired: 14 in]
              }
            }
            n90 = Bundle By Name(cluster=w256, "Core.Last Error.error"=w261) -> (w257:T7)
            n91 = call <vilib>:"Add State(s) to Queue__jki_lib_state_machine.vi"("State(s) in Front (\"\")"=w255, "State(s) in (\"\")"=w266) -> ("States Out"=w265:string)  [unwired: 13 in]
          }
          frame "Macro: Run Sequence" {
            # "0,1,2,3,4,"
            # "5"
            # "Do not put any code in this frame.\n(It is a separator no-op. You can make a copy of this frame to create a new Macro frame)"
            n92 = Unbundle By Name(w277) -> ("sequence"=w273:string[], "Running Step"=w271:i32)
            n93 = Array Size(array=w273) -> (size(s)=w283:i32)
            n94 = Index Array(array=w273, index=w271) -> (element=w272:string)
            n95 = Greater Or Equal?(x=w283, y=w271) -> (x >= y?=w275:bool)
            n96 = Select(t=-1 ("Running Step"), s=w275, f=w271) -> (s? t:f=w282:i32)
            n97 = Bundle By Name(cluster=w277, "Running Step"=w282) -> (w278:T7)
            n98 = Select(t="Sequence: Status >> ...", s=w275, f="Idle //Check Event Structure\nMacro: Run Sequence" ("State(s) at Back (\"\")")) -> (s? t:f=w274:string)
            n99 = call <vilib>:"Add State(s) to Queue__jki_lib_state_machine.vi"("State(s) in Front (\"\")"=w272, "State(s) at Back (\"\")"=w274) -> ("States Out"=w276:string)  [unwired: 13 in]
            n100 = call <vilib>:"Add State(s) to Queue__jki_lib_state_machine.vi"("State(s) in Front (\"\")"=w276, "State(s) in (\"\")"=w287) -> ("States Out"=w286:string)  [unwired: 13 in]
          }
          frame "Macro: Exit" {
            # "Exit Macro\n(This is called once, when the VI exits)"
            n101 = Unbundle By Name(w291) -> ("Core.Close Panel on Exit?"=w289:bool)
            n102 = Bundle By Name(cluster=w291, "Core.Shutdown?"=TRUE) -> (w288:T7)
            n103 = Select(t="UI: Front Panel State >> Close", s=w289, f="" ("Empty String Constant")) -> (s? t:f=w301:string)
            n104 = call <vilib>:"Add State(s) to Queue__jki_lib_state_machine.vi"("State(s) in Front (\"\")"="Data: Cleanup\nEvents: Unregister", "State(s) in (\"\")"="Process: Sync", "State(s) at Back (\"\")"="Exit") -> ("States Out"=w296:string)  [unwired: 12 in]
            n105 = call <vilib>:"Add State(s) to Queue__jki_lib_state_machine.vi"("State(s) in Front (\"\")"="Instrument: Close Hardware", "State(s) in (\"\")"=w301, "State(s) at Back (\"\")"=w296) -> ("States Out"=w300:string)  [unwired: 12 in]
            n106 = call <vilib>:"Add State(s) to Queue__jki_lib_state_machine.vi"("State(s) in Front (\"\")"=w300, "State(s) in (\"\")"=w304) -> ("States Out"=w303:string)  [unwired: 13 in]
          }
          frame "---------- Process ----------" {
            # "Template Separator\n(You can make a copy of, or modify, this frame)"
            n107 = call <vilib>:"Add State(s) to Queue__jki_lib_state_machine.vi"("State(s) in (\"\")"=w309) -> ("States Out"=w308:string)  [unwired: 14 in]
          }
          frame "Process: Sync" {
            n108 = Unbundle By Name(w317) -> ("SMO"=w313:refnum<class "Inst.Xeryon-Rotator.lvclass">)
            n109 = call <vilib>:"WaitOnProcessSync.vi"("error in (no error)"=w312, "SMO"=w313) -> ("error out"=w311:errorcluster, "Don't run?"=w316:bool)  [unwired: 7 in, 1 out]
            n110 = Select(t="Data: Cleanup\nEvents: Unregister\nExit", s=w316, f="" ("Empty String Constant")) -> (s? t:f=w310:string)
            n111 = call <vilib>:"Add State(s) to Queue__jki_lib_state_machine.vi"("State(s) in Front (\"\")"=w310, "State(s) in (\"\")"=w320) -> ("States Out"=w319:string)  [unwired: 13 in]
          }
          frame "---------- Events ----------" {
            # "Template Separator\n(You can make a copy of, or modify, this frame)"
            n112 = call <vilib>:"Add State(s) to Queue__jki_lib_state_machine.vi"("State(s) in (\"\")"=w325) -> ("States Out"=w324:string)  [unwired: 14 in]
          }
          frame "Events: Register" {
            n113 = Unbundle By Name(w331) -> ("SMO"=w332:refnum<class "Inst.Xeryon-Rotator.lvclass">)
            n114 = call <vilib>:"GetProtectedEvents.vi"("SMO"=w332) -> ("error out"=w330:errorcluster, "SMO Protected Events"=w335:T10, "SMO out"=w329:refnum<class "Inst.Xeryon-Rotator.lvclass">)  [unwired: 8 in]
            n115 = call "Inst.Xeryon-Rotator.GetPrivateEvents.vi"("Inst.Xeryon-Rotator in"=w329) -> ("error out"=w326:errorcluster, "Inst.Xeryon-Rotator Private Events"=w327:cluster{"MessageToProcess":refnum<user-event>})  [unwired: 8 in, 1 out]
            n116 = register-events(w335, w327) -> (reference out=w336:refnum<event-registration>, error out=w333:errorcluster)  [unwired: 2 in]
            n117 = Merge Errors(w333, w326, w330, w328) -> (w334:errorcluster)
            n118 = call <vilib>:"Add State(s) to Queue__jki_lib_state_machine.vi"("State(s) in (\"\")"=w338) -> ("States Out"=w337:string)  [unwired: 14 in]
          }
          frame "Events: Unregister" {
            n119 = Unregister For Events(event registration refnum=w341, error in=w340) -> (error out=w339:errorcluster)
            n120 = call <vilib>:"Clear Errors.vi"("error in (no error)"=w339) -> ()  [unwired: 5 in, 2 out]
            n121 = call <vilib>:"Add State(s) to Queue__jki_lib_state_machine.vi"("State(s) in (\"\")"=w344) -> ("States Out"=w343:string)  [unwired: 14 in]
          }
          frame "---------- Instrument ----------" {
            n122 = Unbundle By Name(w346) -> ("SMO"=w345:refnum<class "Inst.Xeryon-Rotator.lvclass">)
            n123 = Bundle By Name(cluster=w346, "SMO"=w345) -> (w347:T7)
            n124 = call <vilib>:"Add State(s) to Queue__jki_lib_state_machine.vi"("State(s) in (\"\")"=w351) -> ("States Out"=w350:string)  [unwired: 14 in]
          }
          frame "Instrument: Open Hardware" {
            n125 = Unbundle By Name(w356) -> ("SMO"=w355:refnum<class "Inst.Xeryon-Rotator.lvclass">)
            n126 = call-dynamic "Open Hardware.vi"("error in (no error)"=w352, "Inst.Xeryon-Rotator in"=w355) -> ("error out"=w353:errorcluster, "Inst.Xeryon-Rotator out"=w354:refnum<class "Inst.Xeryon-Rotator.lvclass">)  [unwired: 8 in]
            n127 = Bundle By Name(cluster=w356, "SMO"=w354) -> (w357:T7)
            n128 = call <vilib>:"Add State(s) to Queue__jki_lib_state_machine.vi"("State(s) in (\"\")"=w360) -> ("States Out"=w359:string)  [unwired: 14 in]
          }
          frame "Instrument: Close Hardware" {
            n129 = Unbundle By Name(w365) -> ("SMO"=w364:refnum<class "Inst.Xeryon-Rotator.lvclass">)
            n130 = call-dynamic "Close Hardware.vi"("error in (no error)"=w361, "Inst.Xeryon-Rotator in"=w364) -> ("error out"=w362:errorcluster, "Inst.Xeryon-Rotator out"=w363:refnum<class "Inst.Xeryon-Rotator.lvclass">)  [unwired: 8 in]
            n131 = Bundle By Name(cluster=w365, "SMO"=w363) -> (w366:T7)
            n132 = call <vilib>:"Add State(s) to Queue__jki_lib_state_machine.vi"("State(s) in (\"\")"=w369) -> ("States Out"=w368:string)  [unwired: 14 in]
          }
          frame "Instrument: GetAll" {
            # "communicate with\nhardware"
            n133 = Unbundle By Name(w379) -> ("SMO"=w378:refnum<class "Inst.Xeryon-Rotator.lvclass">, "MessageToProcess.Message.ID"=w370:string)
            n134 = call "Inst.Xeryon-Rotator.GetAllData.vi"("error in (no error)"=w377, "Inst.Xeryon-Rotator in"=w378) -> ("error out"=w373:errorcluster, "Data out"=w372:variant, "Inst.Xeryon-Rotator out"=w376:refnum<class "Inst.Xeryon-Rotator.lvclass">)  [unwired: 7 in]
            n135 = Empty String/Path?(string/path=w372) -> (empty?=w371:bool)
            n136 = case shown="False" w371 {
              tunnel: w376 -> [w388 w392]
              tunnel: [w387 w392] -> w375
              tunnel: [w385 w391] -> w374
              tunnel: w372 -> [w384 _]
              tunnel: w373 -> [w386 w391]
              tunnel: w370 -> [_ _]
              frame False {
                # "send data to\ninstrument:process.vi"
                n137 = call "To JSON Text.vim"("Anything"=w384) -> ("<JSON>"=w390:string)  [unwired: 9 in, 1 out]
                n138 = call <vilib>:"Pretty Print.vi"("JSON"=w390) -> ("<JSON>"=→"Data":string)  [unwired: 8 in, 2 out]
                n139 = call <userlib>:"setAllData.vi"("error in (no error)"=w386, "AllData"=w384, "Instrument in"=w388) -> ("error out"=w385:errorcluster, "Instrument out"=w387:refnum<class "Inst.Xeryon-Rotator.lvclass">)  [unwired: 7 in]
              }
              frame True {
              }
            }
            n140 = Bundle By Name(cluster=w379, "SMO"=w375) -> (w380:T7)
            n141 = call <vilib>:"Add State(s) to Queue__jki_lib_state_machine.vi"("State(s) in (\"\")"=w383) -> ("States Out"=w382:string)  [unwired: 14 in]
          }
          frame "Instrument: setAngle" {
            n142 = Unbundle By Name(w405) -> ("SMO"=w402:refnum<class "Inst.Xeryon-Rotator.lvclass">, "MessageToProcess.Message.Data"=w399:variant)
            n143 = call "JSON to LVtype.vim"("type"=T3 {"angle"=0.0, "rate"=0.0, "channel"=0} ("setAngle"), "error in (no error)"=w393, "JSON Data in"=w399) -> ("error out"=w394:errorcluster, "Data out"=w397:T3)  [unwired: 7 in]
            n144 = Unbundle By Name(w397) -> ("rate"=w396:dbl, "angle"=w395:dbl)
            n145 = call "Inst.Xeryon-Rotator.Set Speed.vi"("error in (no error)"=w394, "Rate (°/min)"=w396, "Inst.Xeryon-Rotator in"=w402) -> ("error out"=w400:errorcluster, "Inst.Xeryon-Rotator out"=w401:refnum<class "Inst.Xeryon-Rotator.lvclass">)  [unwired: 7 in]
            n146 = call "Inst.Xeryon-Rotator.Set Angle.vi"("error in (no error)"=w400, "Angle (°)"=w395, "Inst.Xeryon-Rotator in"=w401) -> ("error out"=w404:errorcluster, "Inst.Xeryon-Rotator out"=w403:refnum<class "Inst.Xeryon-Rotator.lvclass">)  [unwired: 7 in]
            n147 = Bundle By Name(cluster=w405, "SMO"=w403) -> (w406:T7)
            n148 = call <vilib>:"Add State(s) to Queue__jki_lib_state_machine.vi"("State(s) in (\"\")"=w409) -> ("States Out"=w408:string)  [unwired: 14 in]
          }
          frame "Instrument: setState" {
            n149 = Unbundle By Name(w418) -> ("SMO"=w417:refnum<class "Inst.Xeryon-Rotator.lvclass">, "MessageToProcess.Message.Data"=w414:variant)
            n150 = call "JSON to LVtype.vim"("type"=Inst.Xeryon-Rotator.ScanState--Enum."Stop" ("Scan State"), "error in (no error)"=w412, "JSON Data in"=w414) -> ("error out"=w413:errorcluster, "Data out"=w410:T4)  [unwired: 7 in]
            n151 = call "Inst.Xeryon-Rotator.Set State.vi"("error in (no error)"=w413, "Scan State"=w410, "Inst.Xeryon-Rotator in"=w417) -> ("error out"=w415:errorcluster, "Inst.Xeryon-Rotator out"=w416:refnum<class "Inst.Xeryon-Rotator.lvclass">)  [unwired: 7 in]
            n152 = Bundle By Name(cluster=w418, "SMO"=w416) -> (w419:T7)
            n153 = call <vilib>:"Add State(s) to Queue__jki_lib_state_machine.vi"("State(s) in (\"\")"=w422) -> ("States Out"=w421:string)  [unwired: 14 in]
          }
          frame "Instrument: sendCommand" {
            n154 = Unbundle By Name(w434) -> ("SMO"=w430:refnum<class "Inst.Xeryon-Rotator.lvclass">, "MessageToProcess.Message.Data"=w433:variant)
            n155 = call "JSON to LVtype.vim"("type"="", "error in (no error)"=w432, "JSON Data in"=w433) -> ("error out"=w428:errorcluster, "Data out"=w425:string)  [unwired: 7 in]
            n156 = Match Pattern(string=w425, regular expression="=") -> (before substring=w424:string, after substring=w423:string)  [unwired: 1 in, 2 out]
            n157 = call "Inst.Xeryon-Rotator.sendCommand.vi"("error in (no error)"=w428, "Value"=w423, "Command"=w424, "Inst.Xeryon-Rotator in"=w430) -> ("error out"=w427:errorcluster, "Inst.Xeryon-Rotator out"=w429:refnum<class "Inst.Xeryon-Rotator.lvclass">)  [unwired: 6 in]
            n158 = Bundle By Name(cluster=w434, "SMO"=w429) -> (w435:T7)
            n159 = call <vilib>:"Add State(s) to Queue__jki_lib_state_machine.vi"("State(s) in (\"\")"=w438) -> ("States Out"=w437:string)  [unwired: 14 in]
          }
          frame "Instrument: Log" {
            n160 = Unbundle By Name(w450) -> ("SMO"=w439:refnum<class "Inst.Xeryon-Rotator.lvclass">)
            n161 = call-dynamic "Get SMO Database Paths.vi"("error in (no error)"=w449, "Inst.Xeryon-Rotator in"=w439) -> ("error out"=w447:errorcluster, "Paths"=w448:string, "Inst.Xeryon-Rotator out"=w441:refnum<class "Inst.Xeryon-Rotator.lvclass">)  [unwired: 7 in]
            n162 = Unbundle By Name(w441) -> ("Encoder position [selected units]"=w445:dbl, "Desired Position [selected units]"=w443:dbl, "Status"=w442:string)
            n163 = Bundle("Encoder position [selected units]"=w445, "Desired Position [selected units]"=w443, "Status"=w442) -> (w444:T11)  [unwired: 1 in]
            n164 = call <userlib>:"Instrument.logToDatabase.vi"("error in (no error)"=w447, "Data"=w444, "Paths"=w448, "Instrument"=w441) -> ("error out"=w446:errorcluster, "Instrument out"=w440:refnum<class "Inst.Xeryon-Rotator.lvclass">)  [unwired: 6 in]
            n165 = Bundle By Name(cluster=w450, "SMO"=w440) -> (w451:T7)
            n166 = call <vilib>:"Add State(s) to Queue__jki_lib_state_machine.vi"("State(s) in (\"\")"=w454) -> ("States Out"=w453:string)  [unwired: 14 in]
          }
          frame "---------- Sequence ----------" {
            n167 = call <vilib>:"Add State(s) to Queue__jki_lib_state_machine.vi"("State(s) in (\"\")"=w459) -> ("States Out"=w458:string)  [unwired: 14 in]
          }
          frame "Sequence: Status" {
            # "Sequence: Status\n(Use this frame to pass the status to the UI, this VI's UI, etc)"
            n168 = call <vilib>:"Add State(s) to Queue__jki_lib_state_machine.vi"("State(s) in (\"\")"=w465) -> ("States Out"=w464:string)  [unwired: 14 in]
            "Status" <- w460
          }
          frame "Sequence: Wait" {
            # "Sequence: Wait\n(Non-Blocking Wait)"
            # "F = repeat this state. wait\nT = go to next state. don't wait"
            n169 = Unbundle By Name(w474) -> ("Running Step"=w467:i32)
            n170 = call <userlib>:"Wait Logic.vi"("error in (no error)"=w470, "Time"=w468) -> ("error out"=w469:errorcluster, "Status String"=w466:string, "Trigger"=w471:bool)  [unwired: 6 in, 1 out]
            n171 = Increment(x=w467) -> (x+1=w481:i32)
            n172 = Select(t=w481, s=w471, f=w467) -> (s? t:f=w472:i32)
            n173 = Select(t=u32 0, s=w471, f=u32 100 ("milliseconds to wait")) -> (s? t:f=w478:u32)
            n174 = call <userlib>:"Wait (ms)__ogtk.vi"("error in (no error)"=w469, "milliseconds to wait"=w478) -> ("error out"=w476:errorcluster)  [unwired: 8 in, 1 out]
            n175 = Bundle By Name(cluster=w474, "Running Step"=w472) -> (w473:T7)
            n176 = call <vilib>:"Build State String with Arguments__JKI_lib_State_Machine.vi"("Arguments (\"\")"=w466, "State"="Sequence: Status") -> ("State with Arguments"=w475:string)  [unwired: 4 in]
            n177 = call <vilib>:"Add State(s) to Queue__jki_lib_state_machine.vi"("State(s) in Front (\"\")"=w475, "State(s) in (\"\")"=w484) -> ("States Out"=w483:string)  [unwired: 13 in]
          }
        }
      }
    }
    frame Error {
    }
  }
  n178 = call-parent "Process.vi"("error in"=w5, "Instrument"=w4) -> ("error out"=w2:errorcluster, "Instrument out"=→"Inst.Xeryon-Rotator out":refnum<class "Inst.Xeryon-Rotator.lvclass">)  [unwired: 8 in]
  n179 = Merge Errors(w2, w1) -> (→"error out":errorcluster)
